vi "initializeUI.vi"(8 "error in (no error)":errorcluster, 11 "BuildWorker in":refnum<class "BuildWorker.lvclass">) -> (0 "error out":errorcluster, 3 "BuildWorker out":refnum<class "BuildWorker.lvclass">)   [LabVIEW 2017, in "BuildWorker.lvlib" / "BuildWorker.lvclass"]
uses:
  BuildWorker.lvclass
  C:/Program Files (x86)/National Instruments/LabVIEW 2017/vi.lib/ActorFramework/Actor/Actor.lvclass
  BuildWorker.lvclass/BuildWorker.ctl
  Status.ctl
  <vilib>/ActorFramework/Actor/Actor.lvclass/Actor.ctl
  <vilib>/ActorFramework/Message Enqueuer/Message Enqueuer.lvclass/Message Enqueuer.ctl
  <vilib>/ActorFramework/Message Enqueuer/Init from Existing Queue.vi
  <vilib>/ActorFramework/Message Enqueuer/Message Enqueuer.lvclass
  <vilib>/ActorFramework/Actor/Actor.lvclass
  BuildWorker Messages/Send Worker Status Update Msg/Send Worker Status Update Msg.lvclass
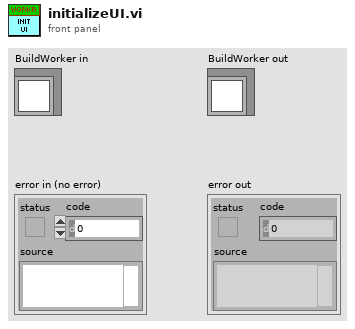
[diagram p1: front panel]
types:
  T1 = typedef "BuildWorker.lvlib/BuildWorker.lvclass/Status.ctl" = enum16{"Created", "Running", "Stopped", "On Error"}
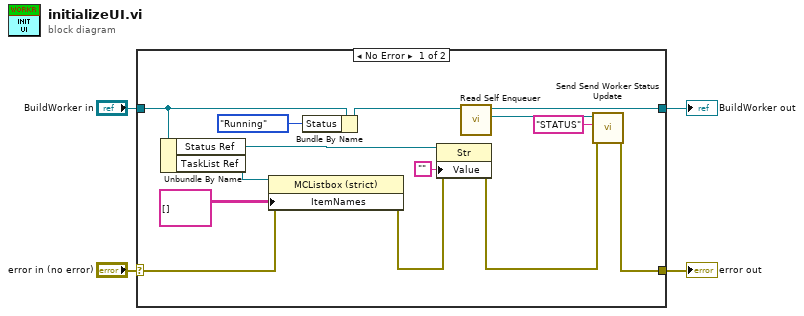
[diagram p0: block diagram]
diagram:
  n1 = case shown="No Error" "error in (no error)" {
    selector: "error in (no error)" -> [w14 w19]
    tunnel: [w9 w19] -> w3
    tunnel: [w7 w18] -> w1
    tunnel: "BuildWorker in" -> [w15 w18]
    frame No Error {
      n2 = Unbundle By Name(w15) -> ("Status Ref"=w13:refnum<vi>, "TaskList Ref"=w17:refnum<vi>)
      n3 = property class="MCListbox (strict)"(reference=w17, error in=w14, "ItemNames"=string[][] [] ("Item Names")) -> (error out=w5:errorcluster)  [unwired: 1 out]
      n4 = Bundle By Name(cluster=w15, "Status"=Status."Running") -> (w7:refnum<class "BuildWorker.lvclass">)
      n5 = property class="Str"(reference=w13, error in=w5, "Value"="") -> (error out=w10:errorcluster)  [unwired: 1 out]
      n6 = call <vilib>:"Read Self Enqueuer.vi"("Actor"=w7) -> ("Self Enqueuer"=w11:refnum<class "Message Enqueuer.lvclass">)  [unwired: 10 in]
      n7 = call "Send Send Worker Status Update.vi"("error in (no error)"=w10, "Operation"="STATUS", "Message Enqueuer in"=w11) -> ("error out"=w9:errorcluster)  [unwired: 7 in, 1 out]
    }
    frame Error {
    }
  }
  "error out" <- w3
  "BuildWorker out" <- w1
